vi "Dispose Array of Images.vi"(0 "Array of Images":T1[](array[typedef]), 3 "error in (no error)":errorcluster) -> (9 "error out":errorcluster)   [LabVIEW 2021, in "Image.lvlib"]
uses:
  Image.lvlib
  <vilib>/vision/Image Controls.llb/IMAQ Image.ctl
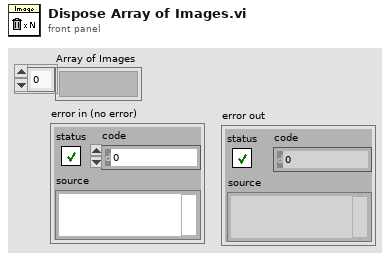
[diagram p1: front panel]
types:
  T1 = typedef "IMAQ Image.ctl" = refnum<image>
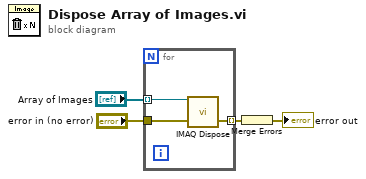
[diagram p0: block diagram]
diagram:
  n1 = for {
    tunnel: "Array of Images" -> [w7] mode=indexing
    tunnel: [w6] -> w3 mode=indexing
    tunnel: "error in (no error)" -> [w5]
    n2 = call "IMAQ Dispose"("Image"=w7, "error in (no error)"=w5) -> ("error out"=w6:errorcluster)  [unwired: 4 in]
  }
  n3 = Merge Errors(w3) -> (→"error out":errorcluster)
